vi "Create.vi"(8 "Error In":errorcluster, 10 "ICommunicate":refnum<class "ICommunicate.lvclass">) -> (0 "Error Out":errorcluster, 3 "SDO Manager":refnum<class "SDO Manager.lvclass">)   [LabVIEW 2020, in "CANopen.lvlib" / "SDO Manager.lvlib" / "SDO Manager.lvclass"]
uses:
  SDO Manager.lvclass
  HAL/Source/Interfaces/ICommunicate/ICommunicate.lvclass
  SDO Manager.lvclass/SDO Manager.ctl
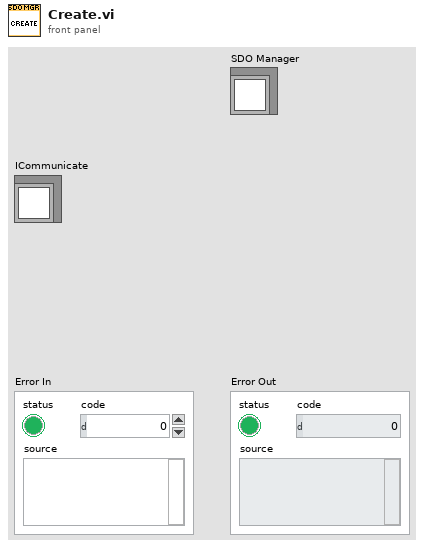
[diagram p1: front panel]
types:
  T1 = typedef "Semaphore RefNum" = refnum<k1>
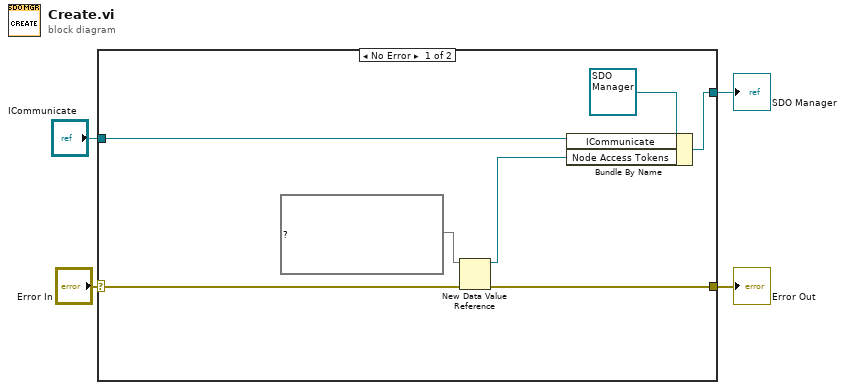
[diagram p0: block diagram]
diagram:
  n1 = case shown="No Error" "Error In" {
    selector: "Error In" -> [w6 w12]
    tunnel: [w9 w12] -> w3
    tunnel: [w10 _] -> w2
    tunnel: "ICommunicate" -> [w7 _]
    frame No Error {
      n2 = New Data Value Reference(data value=map{u8, T1} {} ("Node Access Tokens"), error in=w6) -> (data value reference=w8:refnum<data-value>, error out=w9:errorcluster)
      n3 = Bundle By Name(cluster=refnum<class "SDO Manager.lvclass"> refnum ("reference out"), "ICommunicate"=w7, "Node Access Tokens"=w8) -> (w10:refnum<class "SDO Manager.lvclass">)
    }
    frame Error {
      # "VI-TechBaseTemplate_Simple_4x4x4"
    }
  }
  "Error Out" <- w3
  "SDO Manager" <- w2
